vi "Send Msg To Worker.vi"(8 "error in (no error)":errorcluster, 9 "Message":string, 10 "index":i32, 11 "Comm Interface in":refnum<class "Comm Interface.lvclass">) -> (0 "error out":errorcluster, 3 "Comm Interface out":refnum<class "Comm Interface.lvclass">)   [LabVIEW 2017, in "Comm Interface.lvlib" / "Comm Interface.lvclass"]
uses:
  Comm Interface.lvclass
  Comm Interface.lvclass/Comm Interface.ctl
  WebSocket Server/Actors/Connection Listener/Connection Listener Messages/Forward Message Msg/Forward Message Msg.lvclass/Forward Message Msg.ctl
  <vilib>/ActorFramework/Message Enqueuer/Message Enqueuer.lvclass/Message Enqueuer.ctl
  <vilib>/ActorFramework/Message Enqueuer/Enqueue.vi
  WebSocket Server/Actors/Connection Listener/Connection Listener Messages/Forward Message Msg/Forward Message Msg.lvclass
  Applications/National Instruments/LabVIEW 2017 64-bit/vi.lib/ActorFramework/Message/Message.lvclass
  <vilib>/ActorFramework/Message Priority Queue/Priority Enqueue.vi
  WebSocket Server/Actors/Connection Listener/Connection Listener Messages/Get Connection List Msg/Get Connection List Msg.lvclass
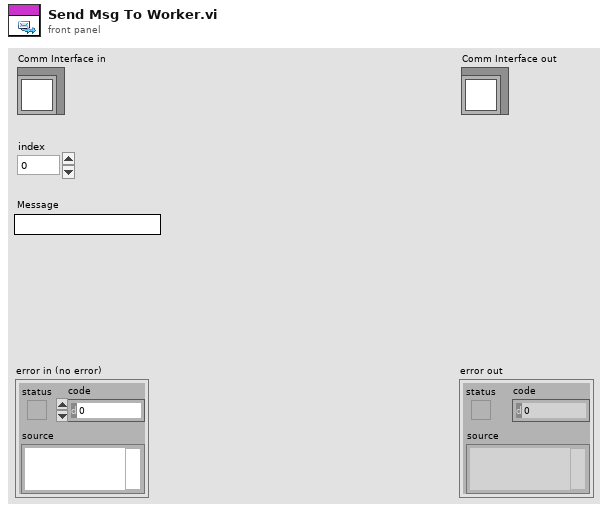
[diagram p1: front panel]
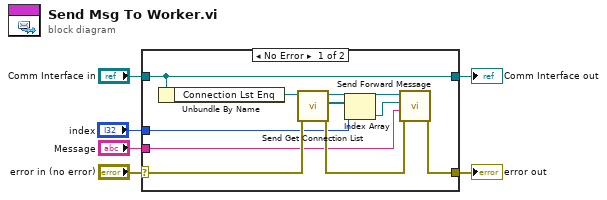
[diagram p0: block diagram]
diagram:
  n1 = case shown="No Error" "error in (no error)" {
    selector: "error in (no error)" -> [w10 w18]
    tunnel: [w11 w18] -> w5
    tunnel: [w12 w17] -> w3
    tunnel: "Comm Interface in" -> [w12 w17]
    tunnel: "Message" -> [w8 _]
    tunnel: "index" -> [w7 _]
    frame No Error {
      n2 = Unbundle By Name(w12) -> ("Connection Lst Enq"=w14:refnum<class "Message Enqueuer.lvclass">)
      n3 = call "Send Get Connection List.vi"("error in (no error)"=w10, "Message Enqueuer in"=w14) -> ("error out"=w9:errorcluster, "Connection List"=w13:refnum<class "Message Enqueuer.lvclass">[], "Message Enqueuer out"=w15:refnum<class "Message Enqueuer.lvclass">)  [unwired: 7 in]
      n4 = Index Array(array=w13, index=w7) -> (element=w16:refnum<class "Message Enqueuer.lvclass">)
      n5 = call "Send Forward Message.vi"("error in (no error)"=w9, "Message"=w8, "Dest Enqueuer"=w16, "Message Enqueuer in"=w15) -> ("error out"=w11:errorcluster)  [unwired: 6 in, 1 out]
    }
    frame Error {
    }
  }
  "error out" <- w5
  "Comm Interface out" <- w3
